vi "Generic_setup.vi"(1 "Setup String":string) -> (0 "Output String":string)   [LabVIEW 2020]
uses:
  Globals/Calib_global.vi
  Controls/ok_button.ctl
panel:
  in  "OK":T1
  in  "Generic Instrument setup":T2
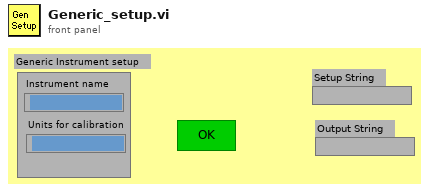
[diagram p1: front panel]
types:
  T1 = typedef "ok_button.ctl" = bool
  T2 = cluster{"Instrument name":string, "Units for calibration":string}
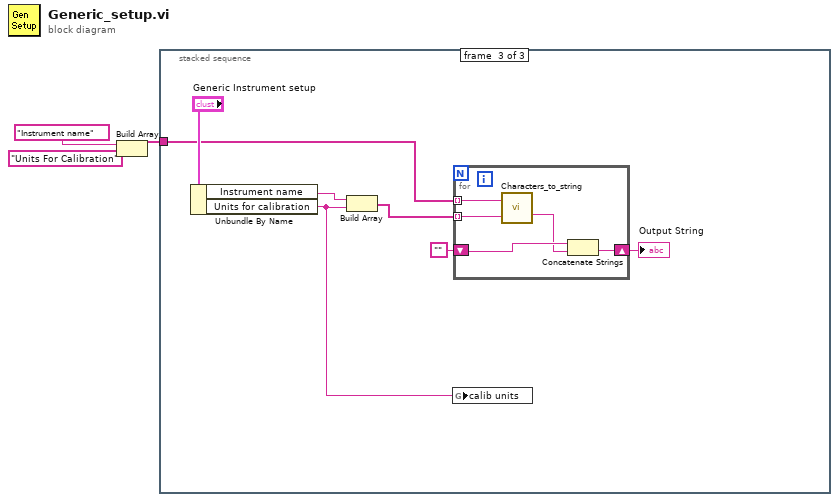
[diagram p0: block diagram]
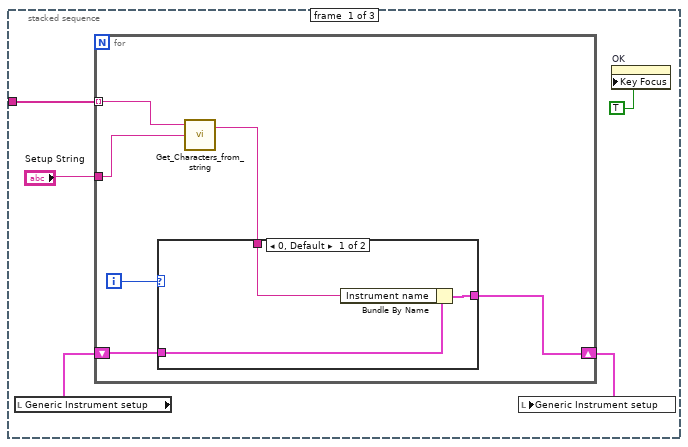
[diagram p2: hidden frame]
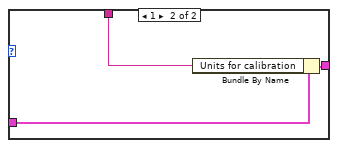
[diagram p3: hidden frame]
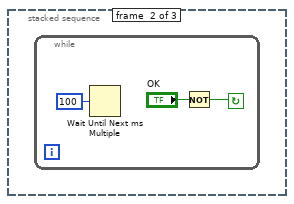
[diagram p4: hidden frame]
diagram:
  n1 = Build Array("Instrument name", "Units For Calibration") -> (w1:string[])
  n2 = stacked-sequence {
    tunnel: w1 -> [w5 _ w25]
    frame #0 {
      n3 = local read "Generic Instrument setup"() -> (w8:T2)
      n4 = for {
        shift-right: [w12] -> w7
        shift-left: w8 -> [w13]
        tunnel: "Setup String" -> [w10]
        tunnel: w5 -> [w11] mode=indexing
        i -> [w14]
        n5 = call "Get_Characters_from_string.vi"("Input string"=w10, "Variable name"=w11) -> ("Value"=w9:string)  [unwired: 1 in, 1 out]
        n6 = case shown="0, Default" w14 {
          tunnel: w13 -> [w17 w20]
          tunnel: [w16 w19] -> w12
          tunnel: w9 -> [w15 w18]
          frame 0, Default {
            n7 = Bundle By Name(cluster=w17, "Instrument name"=w15) -> (w16:T2)
          }
          frame 1 {
            n8 = Bundle By Name(cluster=w20, "Units for calibration"=w18) -> (w19:T2)
          }
        }
      }
      n9 = local write "Generic Instrument setup"(w7) -> ()
      n10 = property on="OK" class="Bool"("Key Focus"=TRUE ("Visible")) -> ()  [unwired: 2 in, 2 out]
    }
    frame #1 {
      n11 = while {
        stop <- w22 continue-if-true
        n12 = Wait Until Next ms Multiple(millisecond multiple=u32 100) -> ()  [unwired: 1 out]
        n13 = Not(x="OK") -> (.not. x?=w22:T1)
      }
    }
    frame #2 {
      n14 = Unbundle By Name("Generic Instrument setup") -> ("Instrument name"=w28:string, "Units for calibration"=w27:string)
      n15 = Build Array(w28, w27) -> (w26:string[])
      n16 = global write "Calib_global.vi" "calib units"(w27) -> ()
      n17 = for {
        shift-right: [w31] -> w24
        shift-left: "" -> [w33]
        tunnel: w25 -> [w35] mode=indexing
        tunnel: w26 -> [w34] mode=indexing
        n18 = call "Characters_to_string.vi"("Characters to write"=w34, "Label for characters"=w35) -> ("Output string"=w32:string)  [unwired: 1 in]
        n19 = Concatenate Strings(w33, w32) -> (w31:string)
      }
      "Output String" <- w24
    }
  }
